vi "To Center and Span.vi"   [LabVIEW 2012]
doc: "Takes two numbers (can have units) that indicate the beginning and end of a range and returns the average (\"center\") and difference (\"span\") of the two numbers."
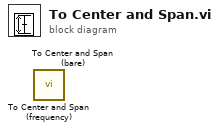
[diagram p0: block diagram]
diagram:
  n1 = call "To Center and Span (frequency).vi"() -> ()  [unwired: 6 in, 2 out]
  n2 = call "To Center and Span (bare).vi"() -> ()  [unwired: 6 in, 2 out]
